vi "remove bad data.vi"(3 "file path":path) -> (0 "size(s)":i32, 1 "text 2":string[](array[string]))   [LabVIEW 2018]
panel:
  out "text":string[](array[string])
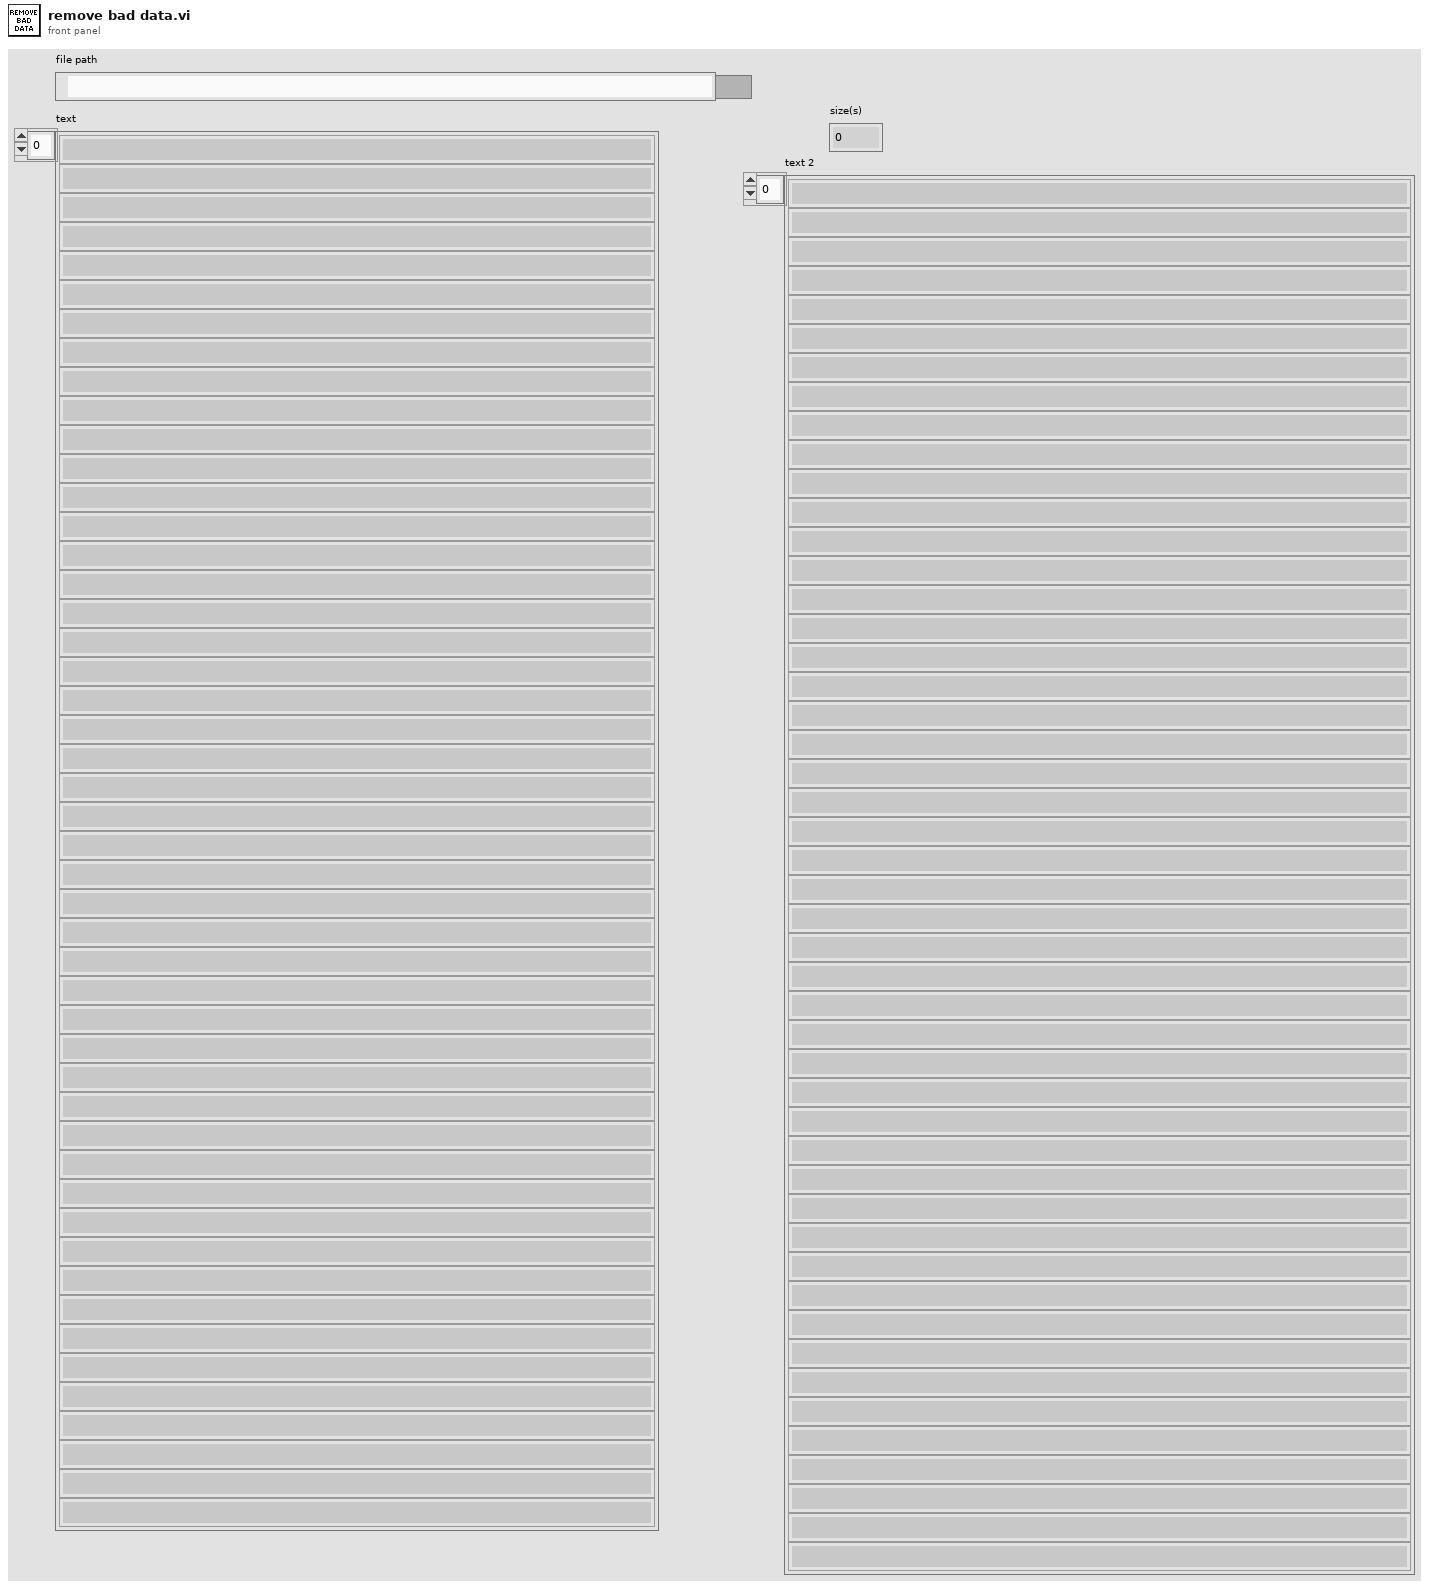
[diagram p1: front panel]
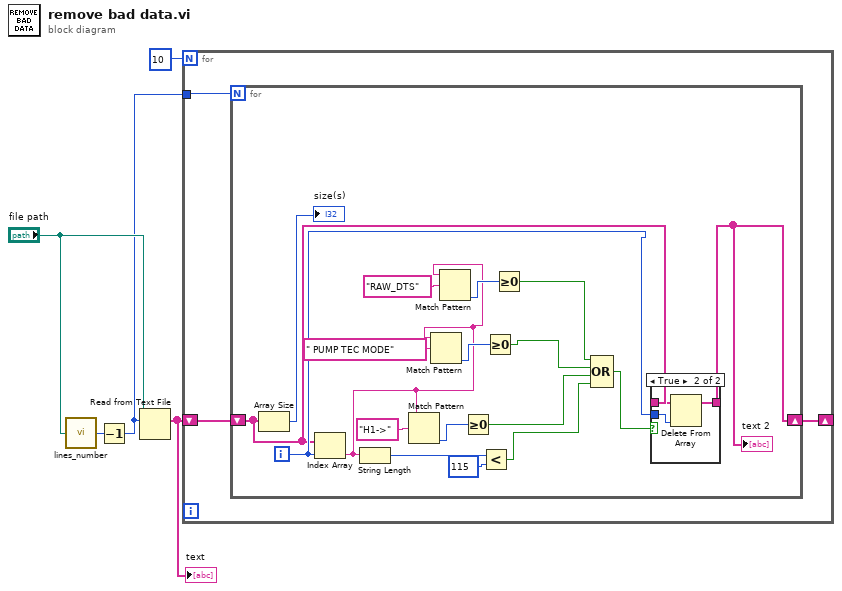
[diagram p0: block diagram]
diagram:
  n1 = call "lines_number.vi"("file path"="file path") -> ("No. lines"=w4:i32)
  n2 = Decrement(x=w4) -> (x-1=w1:i32)
  n3 = Read from Text File(file (use dialog)="file path", count=w1) -> (text=w2:string[])  [unwired: 2 in, 3 out]
  "text" <- w2
  n4 = for {
    N: 10 -> [_]
    tunnel: w1 -> [w8]
    shift-right: [w6] -> _
    shift-left: w2 -> [w7]
    n5 = for {
      N: w8 -> [_]
      shift-right: [w21] -> w6
      shift-left: w7 -> [w23]
      i -> [w24]
      n6 = Array Size(array=w23) -> (size(s)=→"size(s)":i32)
      n7 = Index Array(array=w23, index=w24) -> (element=w10:string)
      n8 = String Length(string=w10) -> (length=w26:i32)
      n9 = Match Pattern(string=w10, regular expression="H1->") -> (offset past match=w19:i32)  [unwired: 1 in, 3 out]
      n10 = Match Pattern(string=w10, regular expression=" PUMP TEC MODE") -> (offset past match=w17:i32)  [unwired: 1 in, 3 out]
      n11 = Match Pattern(string=w10, regular expression="RAW_DTS") -> (offset past match=w11:i32)  [unwired: 1 in, 3 out]
      n12 = Greater Or Equal To 0?(x=w19) -> (x >= 0?=w15:bool)
      n13 = Less?(x=w26, y=115) -> (x < y?=w14:bool)
      n14 = Greater Or Equal To 0?(x=w17) -> (x >= 0?=w16:bool)
      n15 = Greater Or Equal To 0?(x=w11) -> (x >= 0?=w9:bool)
      n16 = Compound Arithmetic op=OR(w9, w16, w15, w14) -> (w13:bool)
      n17 = case shown="True" w13 {
        tunnel: w23 -> [w27 w30]
        tunnel: w24 -> [_ w29]
        tunnel: [w27 w28] -> w21
        frame False {
        }
        frame True {
          n18 = Delete From Array(array=w30, index=w29) -> (array with subset deleted=w28:string[])  [unwired: 1 in, 1 out]
        }
      }
      "text 2" <- w21
    }
  }
